vi "Get Expected Power.vi"(8 "error in (no error)":errorcluster, 11 "niDTS BT DUT in":refnum<class "niDTS BT Dut.lvclass">) -> (0 "error out":errorcluster, 2 "Expected Power":dbl, 3 "niDTS BT DUT out":refnum<class "niDTS BT Dut.lvclass">)   [LabVIEW 2015, in "niDTS BT.lvlib" / "niDTS BT Dut.lvclass"]
uses:
  niDTS BT Dut.lvclass
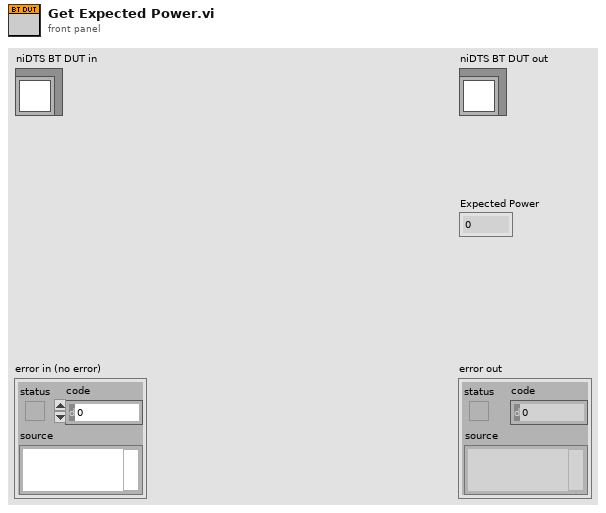
[diagram p1: front panel]
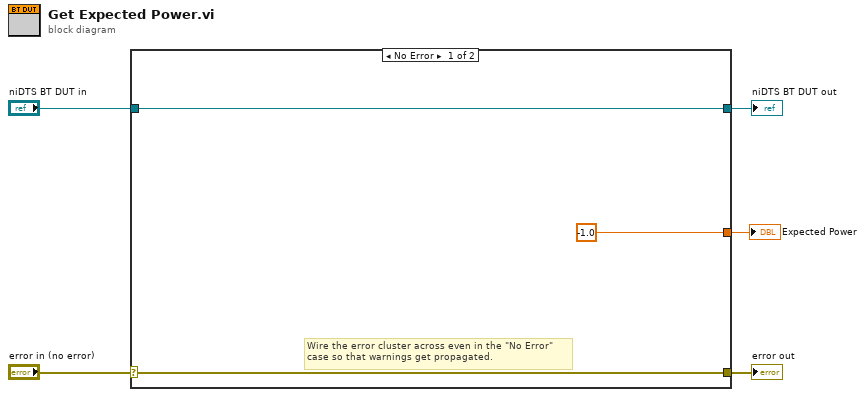
[diagram p0: block diagram]
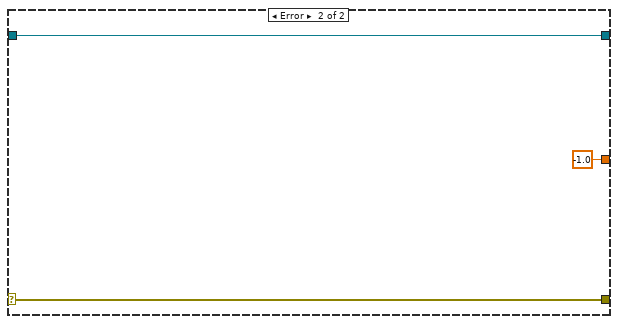
[diagram p2: hidden frame]
diagram:
  n1 = case shown="No Error" "error in (no error)" {
    selector: "error in (no error)" -> [w7 w11]
    tunnel: [w7 w11] -> w4
    tunnel: [w8 w10] -> w2
    tunnel: "niDTS BT DUT in" -> [w8 w10]
    tunnel: [-1.0 -1.0] -> w1
    frame No Error {
      # "Wire the error cluster across even in the \"No Error\"\ncase so that warnings get propagated."
    }
    frame Error {
    }
  }
  "error out" <- w4
  "niDTS BT DUT out" <- w2
  "Expected Power" <- w1
